vi "NI_Read XLSX File.vi"(8 "error in":errorcluster, 11 "XLSX File":path) -> (0 "error out":errorcluster, 2 "Sheet Names":string[](array[string]), 3 "Sheet Data":cluster{"Array":string[][]}[](array[cluster]))   [LabVIEW 2024]
doc: "Reads all sheets from the specified <b>XLSX File</b>. This VI does <b>not</b> require Microsoft Excel to be installed.\n\nEach sheet is returned as a 2D Array of Strings. You will need to perform additional conversion if you require data in numeric format.\n\nTime data (date and/or time) is returned as a number of days elapsed since January 1, 1900. Hour/minute/second information will be returned as a fraction of a day (24 hours)."
uses:
  <vilib>/zip/NI_Unzip.lvlib
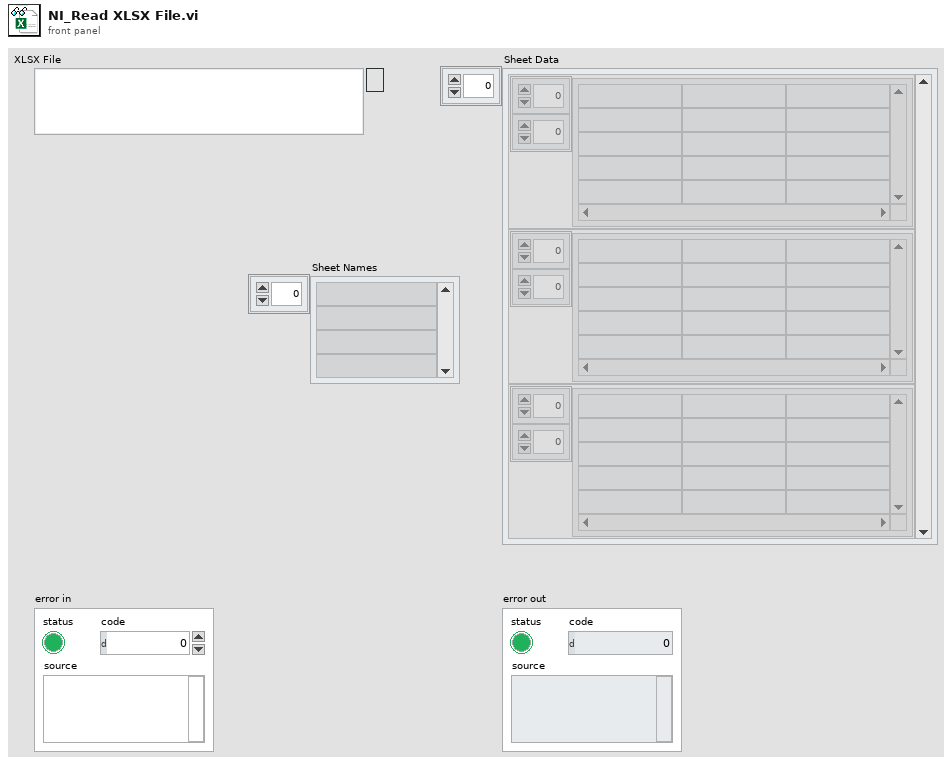
[diagram p1: front panel]
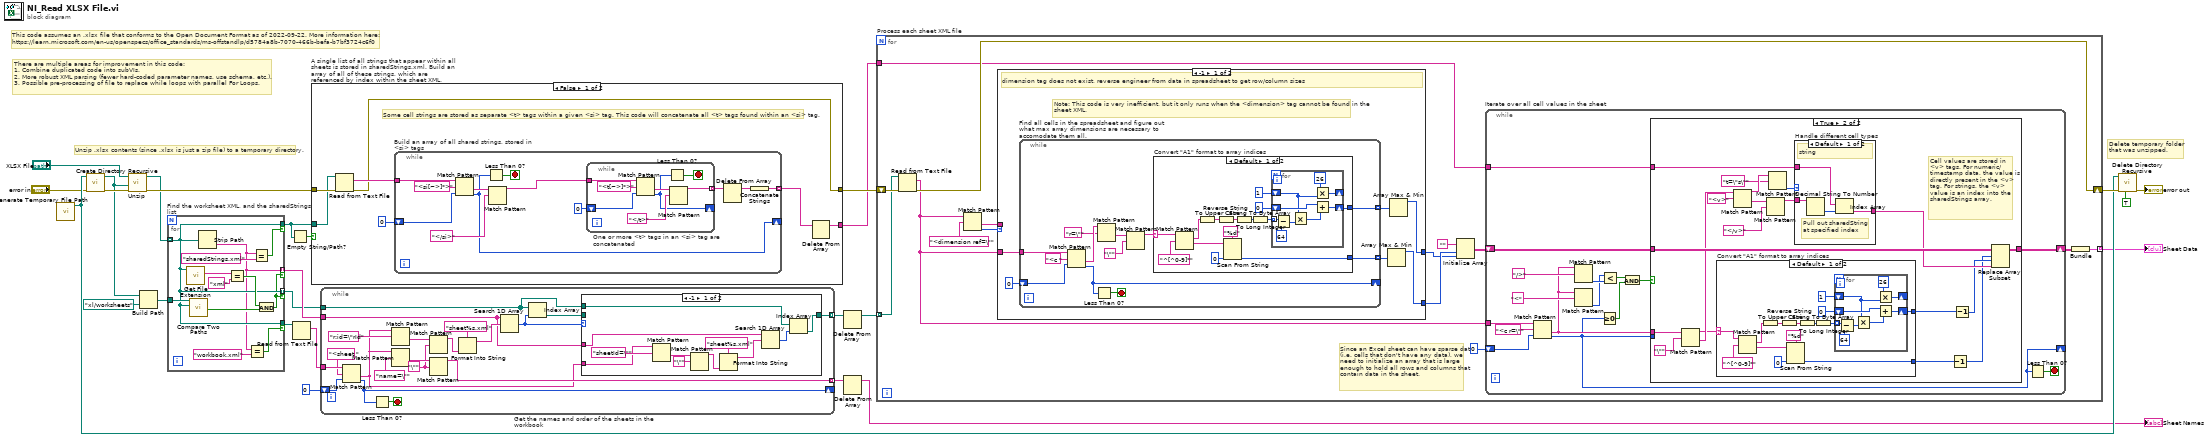
[diagram p0: block diagram]
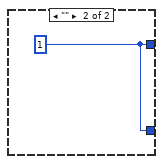
[diagram p4: hidden frame]
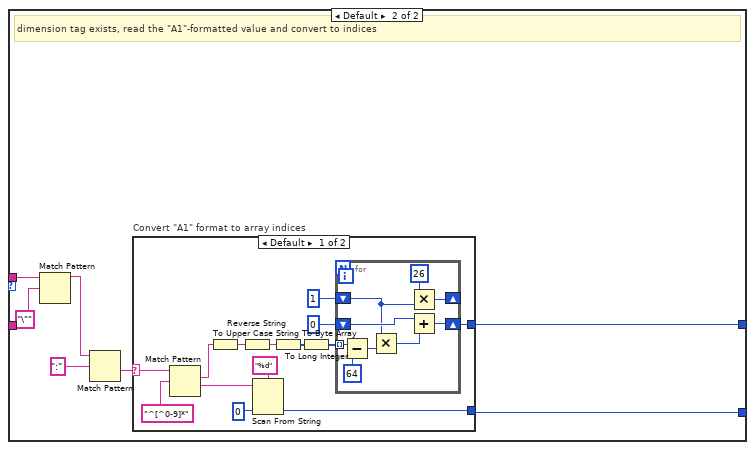
[diagram p5: hidden frame]
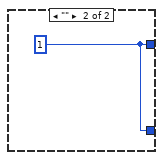
[diagram p6: hidden frame]
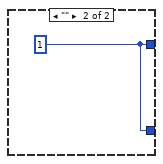
[diagram p8: hidden frame]
diagram:
  # "There are multiple areas for improvement in this code:\n1. Combine duplicated code into subVIs.\n2. More robust XML parsing (fewer hard-coded parameter names, use schema, etc.).\n3. Possible pre-processing of file to replace while loops with parallel For Loops."
  # "Delete temporary folder that was unzipped."
  # "Unzip .xlsx contents (since .xlsx is just a zip file) to a temporary directory."
  # "This code assumes an .xlsx file that conforms to the Open Document Format as of 2022-09-22. More information here:\nhttps://learn.microsoft.com/en-us/openspecs/office_standards/ms-offstandlp/d5784a8b-7070-466b-befa-b7bf3724c6f0"
  n1 = call <vilib>:"Generate Temporary File Path.vi"() -> ("Unique Temporary File Path"=w16:path)  [unwired: 10 in, 1 out]
  n2 = call <vilib>:"Create Directory Recursive.vi"("error in (no error)"="error in", "directory"=w16) -> ("error out"=w26:errorcluster, "directory copy"=w19:path)  [unwired: 3 in, 1 out]
  n3 = call <vilib>:"Unzip.vi"("error in (no error)"=w26, "Target directory (same as Zip file if empty)"=w19, "Zip file"="XLSX File") -> ("error out"=w25:errorcluster, "Unzipped files"=w20:path[])  [unwired: 6 in, 1 out]
  n4 = Build Path(base path=w19, name or relative path=path "xl/worksheets") -> (appended path=w17:path)
  n5 = for "Find the worksheet XML, and the sharedStrings list" {
    tunnel: w20 -> [w30] mode=indexing
    tunnel: [w30] -> w12 if=w35
    tunnel: w17 -> [w37]
    tunnel: [w30] -> w6 mode=indexing if=w27
    tunnel: [w30] -> w10 if=w29
    tunnel: [w28] -> w7 mode=indexing if=w27
    n6 = call <vilib>:"Get File Extension.vi"("file"=w30) -> ("lowercase file extension"=w34:string)  [unwired: 6 in, 4 out]
    n7 = call <vilib>:"Compare Two Paths.vi"("Path 2"=w30, "Path 1"=w37) -> ("Path 2 Relative to Path 1?"=w36:bool)  [unwired: 6 in, 3 out]
    n8 = Strip Path(path=w30) -> (name=w28:string)  [unwired: 1 out]
    n9 = Equal?(x=w34, y="xml") -> (x = y?=w32:bool)
    n10 = Equal?(x=w28, y="workbook.xml") -> (x = y?=w29:bool)
    n11 = Equal?(x=w28, y="sharedStrings.xml") -> (x = y?=w35:bool)
    n12 = And(x=w32, y=w36) -> (x .and. y?=w27:bool)
  }
  n13 = Empty String/Path?(string/path=w12) -> (empty?=w11:bool)
  n14 = Read from Text File(file (use dialog)=w10) -> (text=w9:string)  [unwired: 3 in, 3 out]
  n15 = case "A single list of all strings that appear within all sheets is stored in sharedStrings.xml. Build an array of all of these strings, which are referenced by index within the sheet XML." shown="False" w11 {
    tunnel: w25 -> [w45 w66]
    tunnel: [w40 w66] -> w24
    tunnel: w12 -> [w44 _]
    tunnel: [w41 _] -> w14
    frame False {
      # "Some cell strings are stored as separate <t> tags within a given <si> tag. This code will concatenate all <t> tags found within an <si> tag."
      n16 = Read from Text File(file (use dialog)=w44, error in=w45) -> (text=w43:string, error out=w40:errorcluster)  [unwired: 2 in, 2 out]
      n17 = while "Build an array of all shared strings, stored in <si> tags" {
        tunnel: w43 -> [w49]
        tunnel: [w54] -> w42 mode=indexing
        shift-right: [w48] -> _
        shift-left: 0 -> [w50]
        stop <- w46 stop-if-true
        n18 = Match Pattern(string=w49, regular expression="<si[~>]*>", offset (0)=w50) -> (after substring=w52:string, offset past match=w48:i32)  [unwired: 2 out]
        n19 = Less Than 0?(x=w48) -> (x < 0?=w46:bool)
        n20 = Match Pattern(string=w52, regular expression="</si>") -> (before substring=w47:string)  [unwired: 1 in, 3 out]
        n21 = while "One or more <t> tags in an <si> tag are concatenated" {
          tunnel: w47 -> [w65]
          tunnel: [w61] -> w57 mode=indexing
          shift-right: [w59] -> _
          shift-left: 0 ("offset past match") -> [w58]
          stop <- w60 stop-if-true
          n22 = Match Pattern(string=w65, regular expression="<t[~>]*>", offset (0)=w58) -> (after substring=w63:string, offset past match=w59:i32)  [unwired: 2 out]
          n23 = Less Than 0?(x=w59) -> (x < 0?=w60:bool)
          n24 = Match Pattern(string=w63, regular expression="</t>") -> (before substring=w61:string)  [unwired: 1 in, 3 out]
        }
        n25 = Delete From Array(array=w57) -> (array with subset deleted=w55:string[])  [unwired: 2 in, 1 out]
        n26 = Concatenate Strings(w55) -> (w54:string)
      }
      n27 = Delete From Array(array=w42) -> (array with subset deleted=w41:string[])  [unwired: 2 in, 1 out]
    }
    frame True {
      # "No sharedStrings.xml file within .xlsx."
    }
  }
  n28 = while "Get the names and order of the sheets in the workbook" {
    tunnel: w9 -> [w86]
    shift-right: [w84] -> _
    shift-left: 0 -> [w85]
    tunnel: [w78] -> w3 mode=indexing
    tunnel: w7 -> [w69]
    tunnel: w6 -> [w70]
    tunnel: [w72] -> w5 mode=indexing
    stop <- w82 stop-if-true
    w76 = "\"" ("regular expression")
    n29 = Match Pattern(string=w86, regular expression="<sheet ", offset (0)=w85) -> (after substring=w68:string, offset past match=w84:i32)  [unwired: 2 out]
    n30 = Less Than 0?(x=w84) -> (x < 0?=w82:bool)
    n31 = Match Pattern(string=w68, regular expression="r:id=\"rId") -> (after substring=w77:string)  [unwired: 1 in, 3 out]
    n32 = Match Pattern(string=w68, regular expression="name=\"") -> (after substring=w80:string)  [unwired: 1 in, 3 out]
    n33 = Match Pattern(string=w77, regular expression=w76) -> (before substring=w75:string)  [unwired: 1 in, 3 out]
    n34 = Match Pattern(string=w80, regular expression=w76) -> (before substring=w78:string)  [unwired: 1 in, 3 out]
    n35 = Format Into String(format string="sheet%s.xml", w75) -> (resulting string=w73:string)  [unwired: 2 in, 1 out]
    n36 = Search 1D Array(1D array=w69, element=w73) -> (index of element=w67:i32)  [unwired: 1 in]
    n37 = Index Array(array=w70, index=w67) -> (element=w71:path)
    n38 = case shown="-1" w67 {
      tunnel: [w91 w98] -> w72
      tunnel: w71 -> [_ w98]
      tunnel: w70 -> [w90 _]
      tunnel: w69 -> [w89 _]
      tunnel: w68 -> [w87 _]
      frame -1 {
        n39 = Match Pattern(string=w87, regular expression="sheetId=\"") -> (after substring=w96:string)  [unwired: 1 in, 3 out]
        n40 = Match Pattern(string=w96, regular expression="\"") -> (before substring=w95:string)  [unwired: 1 in, 3 out]
        n41 = Format Into String(format string="sheet%s.xml", w95) -> (resulting string=w93:string)  [unwired: 2 in, 1 out]
        n42 = Search 1D Array(1D array=w89, element=w93) -> (index of element=w92:i32)  [unwired: 1 in]
        n43 = Index Array(array=w90, index=w92) -> (element=w91:path)
      }
      frame Default {
      }
    }
  }
  n44 = Delete From Array(array=w5) -> (array with subset deleted=w4:path[])  [unwired: 2 in, 1 out]
  n45 = Delete From Array(array=w3) -> (array with subset deleted=→"Sheet Names":string[])  [unwired: 2 in, 1 out]
  n46 = for "Process each sheet XML file" {
    shift-right: [w112] -> w23
    shift-left: w24 -> [w113]
    tunnel: w4 -> [w111] mode=indexing
    tunnel: [w105] -> w15 mode=indexing
    tunnel: w14 -> [w103]
    # "Since an Excel sheet can have sparse data (i.e. cells that don't have any data), we need to initialize an array that is large enough to hold all rows and columns that contain data in the sheet."
    n47 = Read from Text File(file (use dialog)=w111, error in=w113) -> (text=w99:string, error out=w112:errorcluster)  [unwired: 2 in, 2 out]
    n48 = Match Pattern(string=w99, regular expression="<dimension ref=\"") -> (after substring=w109:string, offset past match=w100:i32)  [unwired: 1 in, 2 out]
    n49 = case shown="-1" w100 {
      tunnel: w109 -> [_ w162]
      tunnel: [w116 w160] -> w102
      tunnel: [w114 w159] -> w101
      tunnel: w99 -> [w119 _]
      frame -1 {
        # "Note: This code is very inefficient, but it only runs when the <dimension> tag cannot be found in the sheet XML."
        # "dimension tag does not exist, reverse engineer from data in spreadsheet to get row/column sizes"
        n50 = while "Find all cells in the spreadsheet and figure out what max array dimensions are necessary to accomodate them all." {
          tunnel: w119 -> [w131]
          tunnel: [w121] -> w117 mode=indexing
          shift-right: [w127] -> _
          shift-left: 0 -> [w128]
          tunnel: [w120] -> w115 mode=indexing
          stop <- w129 stop-if-true
          n51 = Match Pattern(string=w131, regular expression="<c ", offset (0)=w128) -> (after substring=w126:string, offset past match=w127:i32)  [unwired: 2 out]
          n52 = Less Than 0?(x=w127) -> (x < 0?=w129:bool)
          n53 = Match Pattern(string=w126, regular expression="r=\"") -> (after substring=w124:string)  [unwired: 1 in, 3 out]
          n54 = Match Pattern(string=w124, regular expression="\"") -> (before substring=w122:string)  [unwired: 1 in, 3 out]
          n55 = case "Convert \"A1\" format to array indices" shown="Default" w122 {
            selector: w122 -> [w136 _]
            tunnel: [w139 w155] -> w120
            tunnel: [w135 w155] -> w121
            frame Default {
              n56 = Match Pattern(string=w136, regular expression="^[^0-9]*") -> (match substring=w138:string, after substring=w145:string)  [unwired: 1 in, 2 out]
              n57 = To Upper Case(1:w138) -> (0:w140:string)
              n58 = Reverse String(1:w140) -> (0:w142:string)
              n59 = Scan From String(format string="%d" ("Format String"), input string=w145, default 1=0) -> (output 1=w135:i32)  [unwired: 2 in, 3 out]
              n60 = String To Byte Array(string=w142) -> (unsigned byte array=w141:u8[])
              n61 = To Long Integer(number=w141) -> (32bit integer=w137:i32[])
              n62 = for {
                tunnel: w137 -> [w154] mode=indexing
                shift-right: [w152] -> w139
                shift-left: 0 -> [w149]
                shift-right: [w153] -> _
                shift-left: 1 -> [w148]
                n63 = Subtract(x=w154, y=64) -> (x-y=w150:i32)
                n64 = Multiply(x=w148, y=w150) -> (x*y=w151:i32)
                n65 = Multiply(x=26, y=w148) -> (x*y=w153:i32)
                n66 = Add(x=w149, y=w151) -> (x+y=w152:i32)
              }
            }
            frame "" {
              w155 = 1
            }
          }
        }
        n67 = Array Max & Min(array=w117) -> (max value=w116:i32)  [unwired: 3 out]
        n68 = Array Max & Min(array=w115) -> (max value=w114:i32)  [unwired: 3 out]
      }
      frame Default {
        # "Code copied from:\n[LabVIEW 20xx]\\vi.lib\\addons\\_office\\excel.llb\\Excel Get Excel Location.vi"
        # "dimension tag exists, read the \"A1\"-formatted value and convert to indices"
        n69 = Match Pattern(string=w162, regular expression="\"") -> (before substring=w158:string)  [unwired: 1 in, 3 out]
        n70 = Match Pattern(string=w158, regular expression=":") -> (after substring=w156:string)  [unwired: 1 in, 3 out]
        n71 = case "Convert \"A1\" format to array indices" shown="Default" w156 {
          selector: w156 -> [w167 _]
          tunnel: [w170 w186] -> w159
          tunnel: [w166 w186] -> w160
          frame Default {
            n72 = Match Pattern(string=w167, regular expression="^[^0-9]*") -> (match substring=w169:string, after substring=w176:string)  [unwired: 1 in, 2 out]
            n73 = To Upper Case(1:w169) -> (0:w171:string)
            n74 = Reverse String(1:w171) -> (0:w173:string)
            n75 = Scan From String(format string="%d" ("Format String"), input string=w176, default 1=0) -> (output 1=w166:i32)  [unwired: 2 in, 3 out]
            n76 = String To Byte Array(string=w173) -> (unsigned byte array=w172:u8[])
            n77 = To Long Integer(number=w172) -> (32bit integer=w168:i32[])
            n78 = for {
              tunnel: w168 -> [w185] mode=indexing
              shift-right: [w183] -> w170
              shift-left: 0 -> [w180]
              shift-right: [w184] -> _
              shift-left: 1 -> [w179]
              n79 = Subtract(x=w185, y=64) -> (x-y=w181:i32)
              n80 = Multiply(x=w179, y=w181) -> (x*y=w182:i32)
              n81 = Multiply(x=26, y=w179) -> (x*y=w184:i32)
              n82 = Add(x=w180, y=w182) -> (x+y=w183:i32)
            }
          }
          frame "" {
            w186 = 1
          }
        }
      }
    }
    n83 = Initialize Array("", w102, w101) -> (w107:string[][])
    n84 = while "Iterate over all cell values in the sheet" {
      shift-right: [w198] -> w106
      shift-left: w107 -> [w197]
      tunnel: w99 -> [w202]
      shift-right: [w190] -> _
      shift-left: 0 -> [w200]
      tunnel: w103 -> [w196]
      stop <- w199 stop-if-true
      n85 = Match Pattern(string=w202, regular expression="<c r=\"", offset (0)=w200) -> (after substring=w192:string, offset past match=w190:i32)  [unwired: 2 out]
      n86 = Match Pattern(string=w192, regular expression="/>") -> (offset past match=w193:i32)  [unwired: 1 in, 3 out]
      n87 = Match Pattern(string=w192, regular expression="<") -> (offset past match=w191:i32)  [unwired: 1 in, 3 out]
      n88 = Greater Or Equal To 0?(x=w190) -> (x >= 0?=w188:bool)
      n89 = Less?(x=w191, y=w193) -> (x < y?=w189:bool)
      n90 = And(x=w189, y=w188) -> (x .and. y?=w187:bool)
      n91 = case shown="True" w187 {
        tunnel: w192 -> [_ w222]
        tunnel: [w203 w219] -> w198
        tunnel: w197 -> [w203 w220]
        tunnel: w196 -> [_ w209]
        tunnel: w190 -> [_ _]
        frame False {
          # "No more cells found in the sheet XML. Stop the loop."
        }
        frame True {
          # "Cell values are stored in <v> tags. For numeric/timestamp data, the value is directly present in the <v> tag. For strings, the <v> value is an index into the sharedStrings array."
          n92 = Match Pattern(string=w222, regular expression="\"") -> (before substring=w206:string, after substring=w215:string)  [unwired: 1 in, 2 out]
          n93 = case "Convert \"A1\" format to array indices" shown="Default" w206 {
            selector: w206 -> [w227 _]
            tunnel: [w230 w246] -> w205
            tunnel: [w226 w246] -> w204
            frame Default {
              n94 = Match Pattern(string=w227, regular expression="^[^0-9]*") -> (match substring=w229:string, after substring=w236:string)  [unwired: 1 in, 2 out]
              n95 = To Upper Case(1:w229) -> (0:w231:string)
              n96 = Reverse String(1:w231) -> (0:w233:string)
              n97 = Scan From String(format string="%d" ("Format String"), input string=w236, default 1=0) -> (output 1=w226:i32)  [unwired: 2 in, 3 out]
              n98 = String To Byte Array(string=w233) -> (unsigned byte array=w232:u8[])
              n99 = To Long Integer(number=w232) -> (32bit integer=w228:i32[])
              n100 = for {
                tunnel: w228 -> [w245] mode=indexing
                shift-right: [w243] -> w230
                shift-left: 0 -> [w240]
                shift-right: [w244] -> _
                shift-left: 1 -> [w239]
                n101 = Subtract(x=w245, y=64) -> (x-y=w241:i32)
                n102 = Multiply(x=w239, y=w241) -> (x*y=w242:i32)
                n103 = Multiply(x=26, y=w239) -> (x*y=w244:i32)
                n104 = Add(x=w240, y=w242) -> (x+y=w243:i32)
              }
            }
            frame "" {
              w246 = 1
            }
          }
          n105 = Match Pattern(string=w215, regular expression="<v>") -> (before substring=w214:string, after substring=w217:string)  [unwired: 1 in, 2 out]
          n106 = Match Pattern(string=w217, regular expression="</v>") -> (before substring=w210:string)  [unwired: 1 in, 3 out]
          n107 = Match Pattern(string=w214, regular expression="t=\"s\"") -> (offset past match=w212:i32)  [unwired: 1 in, 3 out]
          n108 = case "Handle different cell types" shown="Default" w212 {
            tunnel: [w248 w251] -> w211
            tunnel: w210 -> [w250 w251]
            tunnel: w209 -> [w247 _]
            frame Default {
              # "Pull out sharedString at specified index"
              # "string"
              n109 = Decimal String To Number(string=w250) -> (number=w249:i32)  [unwired: 2 in, 1 out]
              n110 = Index Array(array=w247, index=w249) -> (element=w248:string)
            }
            frame -1 {
              # "Use <v> value"
              # "number/time stamp"
            }
          }
          n111 = Decrement(x=w204) -> (x-1=w207:i32)
          n112 = Decrement(x=w205) -> (x-1=w208:i32)
          n113 = Replace Array Subset(array=w220, new element=w211, index (row)=w207, index (col)=w208) -> (w219:string[][])
        }
      }
      n114 = Less Than 0?(x=w190) -> (x < 0?=w199:bool)
    }
    n115 = Bundle(w106) -> (w105:cluster{string[][]})  [unwired: 1 in]
  }
  "Sheet Data" <- w15
  n116 = call <vilib>:"Delete Directory Recursive.vi"("keep deleting on error? (F)"=TRUE, "error in (no error)"=w23, "Folder to Delete"=w16) -> ("error out"=→"error out":errorcluster)  [unwired: 7 in, 1 out]
